vi "set Data Element.vi"(0 "LVx - Template Command in":refnum<class "Rex - NART - Transmit.lvclass">, 5 "Transmit Config":T1={"Packet Length"=100, "Packet Count"=100, "Data Rate"="1,0,0", "Frequency, MHz"=2412, "Continuous Frames"=FALSE, "TX Power, dB"=30.0}, 11 "error in (no error)":errorcluster) -> (4 "LVx - Template Command out":refnum<class "Rex - NART - Transmit.lvclass">, 15 "error out":errorcluster)   [LabVIEW 2011, in "ART2 Test Panel.lvlib" / "Rex - NART - Transmit.lvclass"]
uses:
  Rex - NART - Transmit.lvclass
  Components/ART2.llb/NART/Controls/Transmit Config.ctl
  Components/ART2.llb/CART/Controls/Data Rates.ctl
  Rex - NART - Transmit.lvclass/Rex - NART - Transmit.ctl
  ART2 Test Panel.lvlib
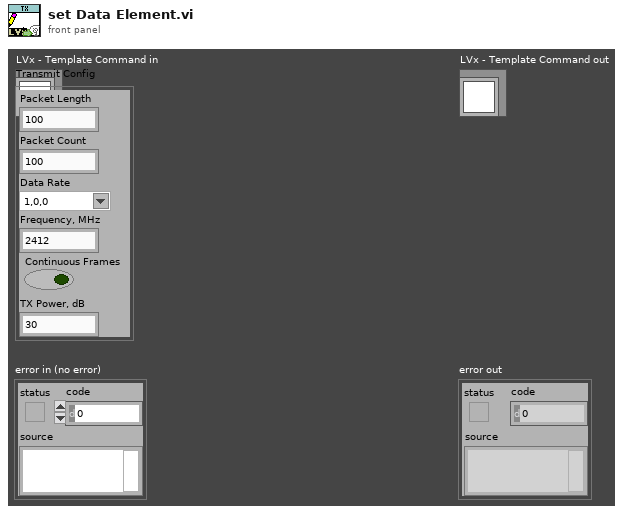
[diagram p1: front panel]
types:
  T1 = typedef "ART2 Test Panel.lvlib/Transmit Config.ctl" = cluster{"Packet Length":u32, "Packet Count":i32, "Data Rate":T2, "Frequency, MHz":u32, "Continuous Frames":bool, "TX Power, dB":dbl}
  T2 = typedef "ART2 Test Panel.lvlib/Data Rates.ctl" = string
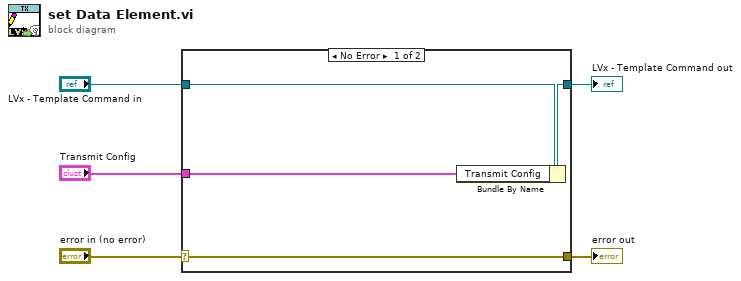
[diagram p0: block diagram]
diagram:
  n1 = case shown="No Error" "error in (no error)" {
    selector: "error in (no error)" -> [w9 w10]
    tunnel: [w9 w10] -> w4
    tunnel: [w7 w11] -> w2
    tunnel: "LVx - Template Command in" -> [w8 w11]
    tunnel: "Transmit Config" -> [w6 _]
    frame No Error {
      n2 = Bundle By Name(cluster=w8, "Transmit Config"=w6) -> (w7:refnum<class "Rex - NART - Transmit.lvclass">)
    }
    frame Error {
    }
  }
  "error out" <- w4
  "LVx - Template Command out" <- w2
